vi "vettore_incompleto.vi"(1 "Lunghezza vettore":u32=11, 2 "Valore massimo":dbl=10.0, 3 "Valore minimo":dbl) -> (0 "Array":dbl[](array[numeric]))   [LabVIEW 2018]
panel:
  out "Waveform Graph":dbl[](graph)
  out "Spaziatura elementi":dbl
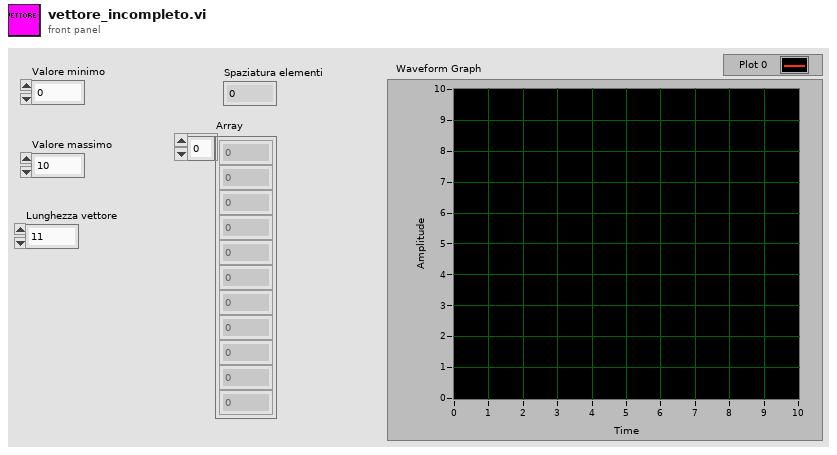
[diagram p1: front panel]
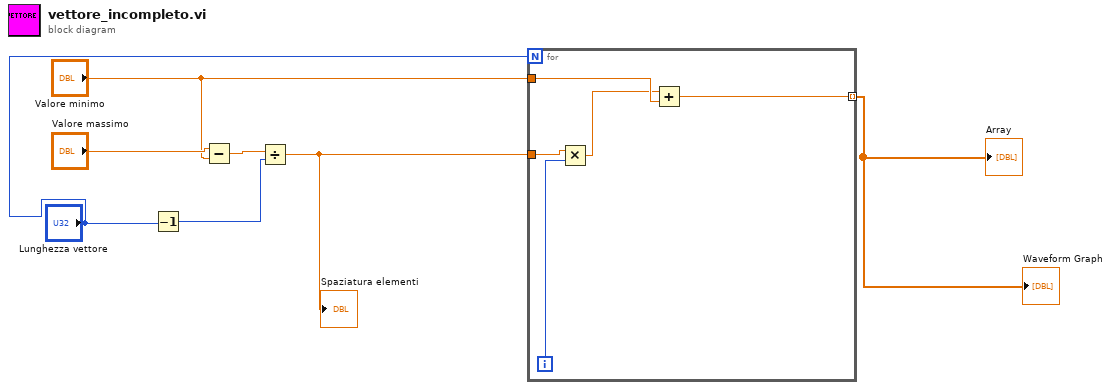
[diagram p0: block diagram]
diagram:
  n1 = Decrement(x="Lunghezza vettore") -> (x-1=w5:u32)
  n2 = Subtract(x="Valore massimo", y="Valore minimo") -> (x-y=w6:dbl)
  n3 = Divide(x=w6, y=w5) -> (x/y=w4:dbl)
  "Spaziatura elementi" <- w4
  n4 = for {
    N: "Lunghezza vettore" -> [_]
    tunnel: w4 -> [w11]
    tunnel: "Valore minimo" -> [w12]
    tunnel: [w8] -> w1 mode=indexing
    i -> [w10]
    n5 = Multiply(x=w11, y=w10) -> (x*y=w9:dbl)
    n6 = Add(x=w9, y=w12) -> (x+y=w8:dbl)
  }
  "Array" <- w1
  "Waveform Graph" <- w1
